vi "Add Subscriber.vi"(8 "error in (no error)":errorcluster, 9 "Message Transport Interface":refnum<class "Message Transport Interface.lvclass">, 10 "Topic Name":string, 11 "Topic Actor in":refnum<class "Topic Actor.lvclass">) -> (0 "error out":errorcluster, 3 "Topic Actor out":refnum<class "Topic Actor.lvclass">)   [LabVIEW 2016, in "Stream Mediator.lvlib" / "Topic Actor.lvclass"]
doc: "--\nCopyright © 2017 Composed SystemsI All rights reserved.\n\nAuthor: Jon McBee <jon.mcbee@composed.io>\n\nThis library is provided \"AS IS\" ,WITHOUT WARRANTIES OR\nCONDITIONS OF ANY KIND, either express or implied.\n\nComposed Systems -- composed.io\n\nStream 0.0.1.1\nJon McBee - Composed Systems\nCopyright (c) 2017, Composed Systems"
uses:
  <userlib>/Composed Systems/Stream/Mediator/Classes/Topic Actor/Topic Actor.lvclass
  <userlib>/Composed Systems/Stream/Mediator/Classes/Message Transport Interface/Message Transport Interface.lvclass
  <userlib>/Composed Systems/Stream/Mediator/Classes/Topic Actor/Topic Actor.lvclass/Topic Actor.ctl
  <userlib>/Composed Systems/Stream/Mediator/Classes/Subscriber Look Up Table/Subscriber Look Up Table.lvclass
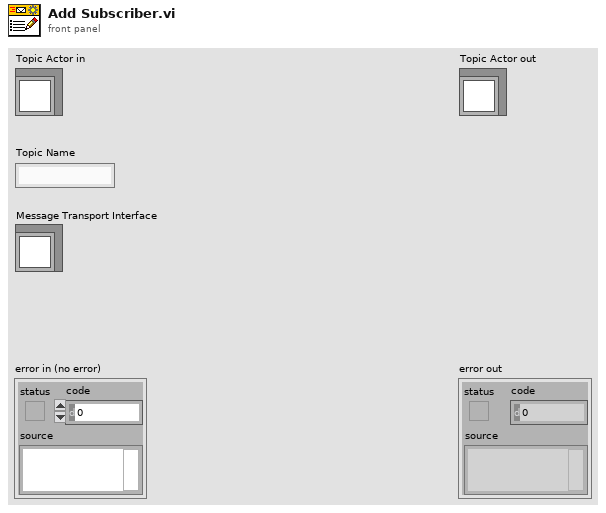
[diagram p1: front panel]
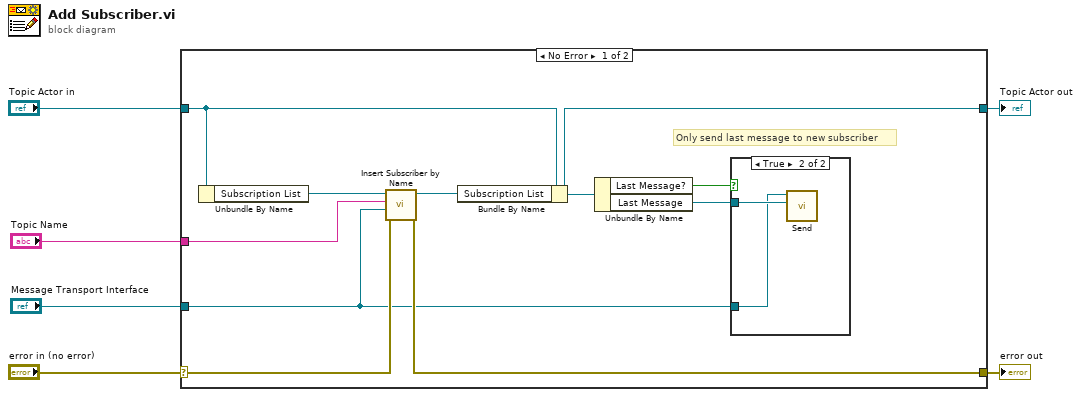
[diagram p0: block diagram]
diagram:
  n1 = case shown="No Error" "error in (no error)" {
    selector: "error in (no error)" -> [w14 w20]
    tunnel: [w13 w20] -> w5
    tunnel: [w10 w19] -> w3
    tunnel: "Topic Actor in" -> [w11 w19]
    tunnel: "Topic Name" -> [w15 _]
    tunnel: "Message Transport Interface" -> [w7 _]
    frame No Error {
      # "Only send last message to new subscriber"
      n2 = Unbundle By Name(w11) -> ("Subscription List"=w16:refnum<class "Subscriber Look Up Table.lvclass">)
      n3 = call <userlib>:"Insert Subscriber by Name.vi"("error in (no error)"=w14, "Subscriber"=w7, "Topic Name"=w15, "Subscriber Index Look Up Table in"=w16) -> ("error out"=w13:errorcluster, "Subscriber Index Look Up Table out"=w12:refnum<class "Subscriber Look Up Table.lvclass">)  [unwired: 5 in, 1 out]
      n4 = Bundle By Name(cluster=w11, "Subscription List"=w12) -> (w10:refnum<class "Topic Actor.lvclass">)
      n5 = Unbundle By Name(w10) -> ("Last Message?"=w9:bool, "Last Message"=w8:refnum<class "Message Interface.lvclass">)
      n6 = case shown="True" w9 {
        tunnel: w8 -> [_ w18]
        tunnel: w7 -> [_ w17]
        frame False {
        }
        frame True {
          n7 = call-dynamic "Send.vi"("Message"=w18, "Message Transport Interface in"=w17) -> ()  [unwired: 7 in, 3 out]
        }
      }
    }
    frame Error {
    }
  }
  "error out" <- w5
  "Topic Actor out" <- w3
